vi "Sub_voltage_read.vi"(4 "error in":errorcluster, 5 "timeout":dbl=10.0 format="%0.2f", 6 "number of samples":i32=100000, 7 "task/channels in":refnum<k21>) -> (0 "error out":errorcluster, 1 "data":dbl[](array[numeric]), 3 "Task out":refnum<k21>)   [LabVIEW 2021]
uses:
  <vilib>/DAQmx/read.llb/DAQmx Read (Analog 1D DBL 1Chan NSamp).vi
  <vilib>/DAQmx/miscellaneous.llb/DAQmx Fill In Error Info.vi
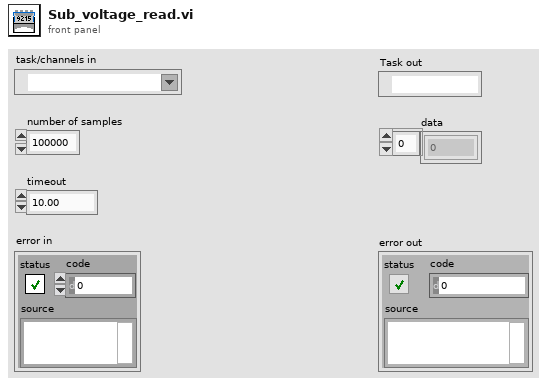
[diagram p1: front panel]
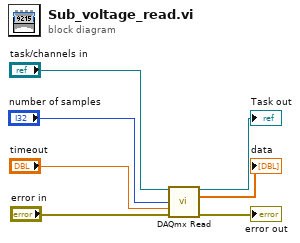
[diagram p0: block diagram]
diagram:
  n1 = call-poly <vilib>:"DAQmx Read.vi"("task/channels in"="task/channels in", "number of samples per channel"="number of samples", "timeout"="timeout", "error in"="error in") -> ("task out"=→"Task out":refnum<k21>, "data"=→"data":dbl[], "error out"=→"error out":errorcluster)  [unwired: 9 in]
